vi "ftp_send_files.vi"(5 "remote folder":string, 7 "Files to move":path[](array[path]), 8 "error in (no error)":errorcluster, 11 "ftp session in":T1) -> (0 "error out":errorcluster, 3 "ftp session out":T1)   [LabVIEW 2017, in "labview-standard-library.lvlib"]
uses:
  <vilib>/FTP/ftp0.llb/FTP Session.ctl
  labview-standard-library.lvlib
  <vilib>/FTP/NI_FTP.lvlib
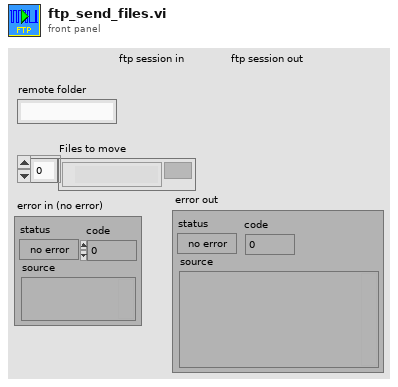
[diagram p1: front panel]
types:
  T1 = typedef "NI_FTP.lvlib/FTP Session.ctl" = refnum<k5>
  T2 = cluster{"remote path":string, "local path":path, "binary":bool, "data":string}
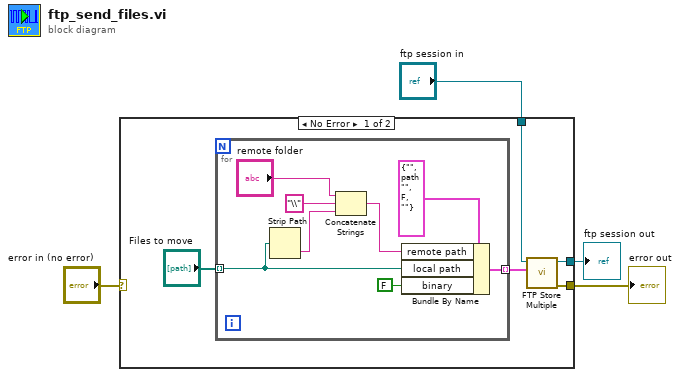
[diagram p0: block diagram]
diagram:
  n1 = case shown="No Error" "error in (no error)" {
    selector: "error in (no error)" -> [_ w19]
    tunnel: [w7 w19] -> w4
    tunnel: "ftp session in" -> [w6 w18]
    tunnel: [w5 w18] -> w1
    frame No Error {
      n2 = for {
        tunnel: [w17] -> w8 mode=indexing
        tunnel: "Files to move" -> [w14] mode=indexing
        n3 = Strip Path(path=w14) -> (name=w13:string)  [unwired: 1 out]
        n4 = Concatenate Strings("remote folder", "\\", w13) -> (w12:string)
        n5 = Bundle By Name(cluster=T2 {"remote path"="", "local path"=path "", "binary"=FALSE, "data"=""} ("transfer spec"), "remote path"=w12, "local path"=w14, "binary"=FALSE) -> (w17:T2)
      }
      n6 = call <vilib>:"FTP Store Multiple.vi"("file specifications"=w8, "ftp session"=w6) -> ("error out"=w7:errorcluster, "ftp session out"=w5:T1)  [unwired: 7 in, 1 out]
    }
    frame Error {
    }
  }
  "error out" <- w4
  "ftp session out" <- w1
